vi "Filter Tester.vi"() -> ()   [LabVIEW 2016]
uses:
  Control/SSL Data Control.ctl
  Control/SSL UDP Address.ctl
  Control/File Player.ctl
  SSL/SSL Field State.ctl
  SSL Detection Frame.ctl
  SSL Detection Robot.ctl
  SSL Detection Ball.ctl
  Filters/Estimadores.ctl
  <extravilib>/ChannelInstances/Lossy Stream-t'SSL Field State.ctl'/Read With Abort.vi
  <extravilib>/ChannelInstances/Lossy Stream-a[.](u8)/Read With Abort.vi
  <extravilib>/ChannelInstances/Lossy Stream-t'SSL Field State.ctl'/Write With Abort.vi
  <extravilib>/ChannelInstances/Lossy Stream-t'SSL Field State.ctl'/Endpoint.vi
  <extravilib>/ChannelInstances/Lossy Stream-a[.](u8)/Endpoint.vi
  <extravilib>/ChannelInstances/Lossy Stream-a[.](u8)/Instantiate.vi
  <extravilib>/ChannelInstances/Lossy Stream-a[.](u8)/)Channel.vi
  <resource>/ChannelSupport/_ChannelSupport/WaitIfNeeded.vi
  <extravilib>/ChannelInstances/Lossy Stream-t'SSL Field State.ctl'/Instantiate.vi
  <extravilib>/ChannelInstances/Lossy Stream-t'SSL Field State.ctl'/)Channel.vi
  <extravilib>/ChannelInstances/Lossy Stream-t'SSL Field State.ctl'.lvlib
  <extravilib>/ChannelInstances/Lossy Stream-a[.](u8).lvlib
panel:
  out "Sinal original":sgl(graph)
  out "Ruido->Kalman":sgl(graph)
  out "Waveform Chart":sgl(graph)
  out "x^2":sgl
  out "Numeric":i32
  out "sum 3":sgl
  out "sum 2":sgl
  out "element":u8[](array[numeric])
  in  "SSL Data":T1={"Modo"=TRUE, "SSL UDP RX"={"Port:"=10020, "Server IP:"="224.5.23.2", "Local IP:"="192.168.91.173", "RX"=TRUE}, "RefBox UDP RX"={"Port:"=10021, "Server IP:"="224.5.23.2", "Local IP:"="192.168.91.173", "RX"=FALSE}, "Reprodução de Arquivo"={"file path (use dialog)"=path "E:/Media/2016-07-01_cmdragons_immortals.log", "size (in bytes)"=0, "offset (in bytes)"=0, "Slide"=0.0, "Play"=FALSE, "Time Stamp"=timestamp(0 s since 1904-01-01), "Playing"=FALSE}} {"Reprodução de Arquivo"."Time Stamp" format="%<%.3X %x>T"; "Reprodução de Arquivo"."Slide" min=0 max=1 scale=0.0..1.0; "Reprodução de Arquivo"."offset (in bytes)" format="%.3p"; "Reprodução de Arquivo"."size (in bytes)" format="%.3p"}
  # "UDP"
  # "LOG"
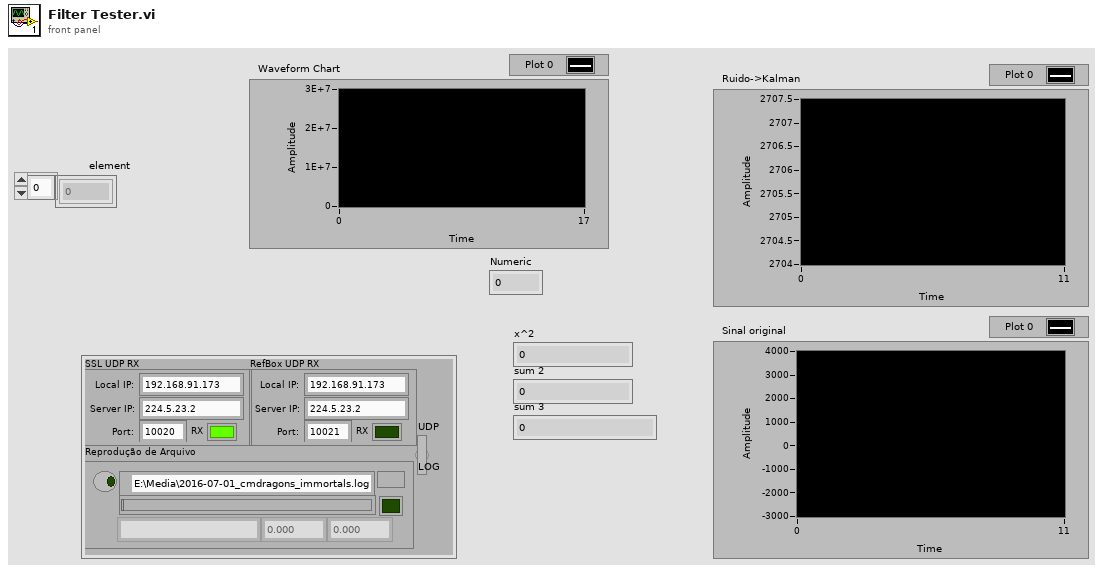
[diagram p1: front panel]
types:
  T1 = typedef "SSL Data Control.ctl" = cluster{"Modo":bool, "SSL UDP RX":T2, "RefBox UDP RX":T2, "Reprodução de Arquivo":T3}
  T2 = typedef "SSL UDP Address.ctl" = cluster{"Port:":u16, "Server IP:":string, "Local IP:":string, "RX":bool}
  T3 = typedef "File Player.ctl" = cluster{"file path (use dialog)":path, "size (in bytes)":i64, "offset (in bytes)":i64, "Slide":sgl, "Play":bool, "Time Stamp":timestamp, "Playing":bool}
  T4 = typedef "Lossy Stream-a[.](u8).lvlib/)Channel.ctl" = refnum<queue>
  T5 = typedef "Estimadores.ctl" = enum16{"Nenhum", "Simples", "Simples Timestamp", "Simples Mult Cam", "Kalman", "Kalman Mult Cam"}
  T6 = typedef "SSL Field State.ctl" = cluster{"Detection Frame Out":T7, "Field Size Out":cluster{"line_width":u32, "field_length":u32, "field_width":u32, "boundary_width":u32, "referee_width":u32, "goal_width":u32, "goal_depth":u32, "goal_wall_width":u32, "center_circle_radius":u32, "defense_radius":u32, "defense_stretch":u32, "free_kick_from_defense_dist":u32, "penalty_spot_from_field_line_dist":u32, "penalty_line_from_spot_dist":u32}, "Received Time Stamp":timestamp}
  T7 = typedef "SSL Detection Frame.ctl" = cluster{"frame_number":u32, "t_capture":dbl, "t_sent":dbl, "camera_id":u32, "robots_yellow":T8[], "robots_blue":T8[], "balls":T9[], "Valid":bool, "Time Stamp":timestamp}
  T8 = typedef "SSL Detection Robot.ctl" = cluster{"x":sgl, "robot_id":u32, "confidence":sgl, "y":sgl, "orientation":sgl, "pixel_x":sgl, "pixel_y":sgl, "height":sgl, "Valid":bool, "Time Stamp":timestamp}
  T9 = typedef "SSL Detection Ball.ctl" = cluster{"x":sgl, "area":u32, "confidence":sgl, "y":sgl, "z":sgl, "pixel_x":sgl, "pixel_y":sgl, "Valid":bool, "Time Stamp":timestamp}
  T10 = cluster{"line_width":u32, "field_length":u32, "field_width":u32, "boundary_width":u32, "referee_width":u32, "goal_width":u32, "goal_depth":u32, "goal_wall_width":u32, "center_circle_radius":u32, "defense_radius":u32, "defense_stretch":u32, "free_kick_from_defense_dist":u32, "penalty_spot_from_field_line_dist":u32, "penalty_line_from_spot_dist":u32}
  T11 = typedef "Lossy Stream-t'SSL Field State.ctl'.lvlib/)Channel.ctl" = refnum<queue>
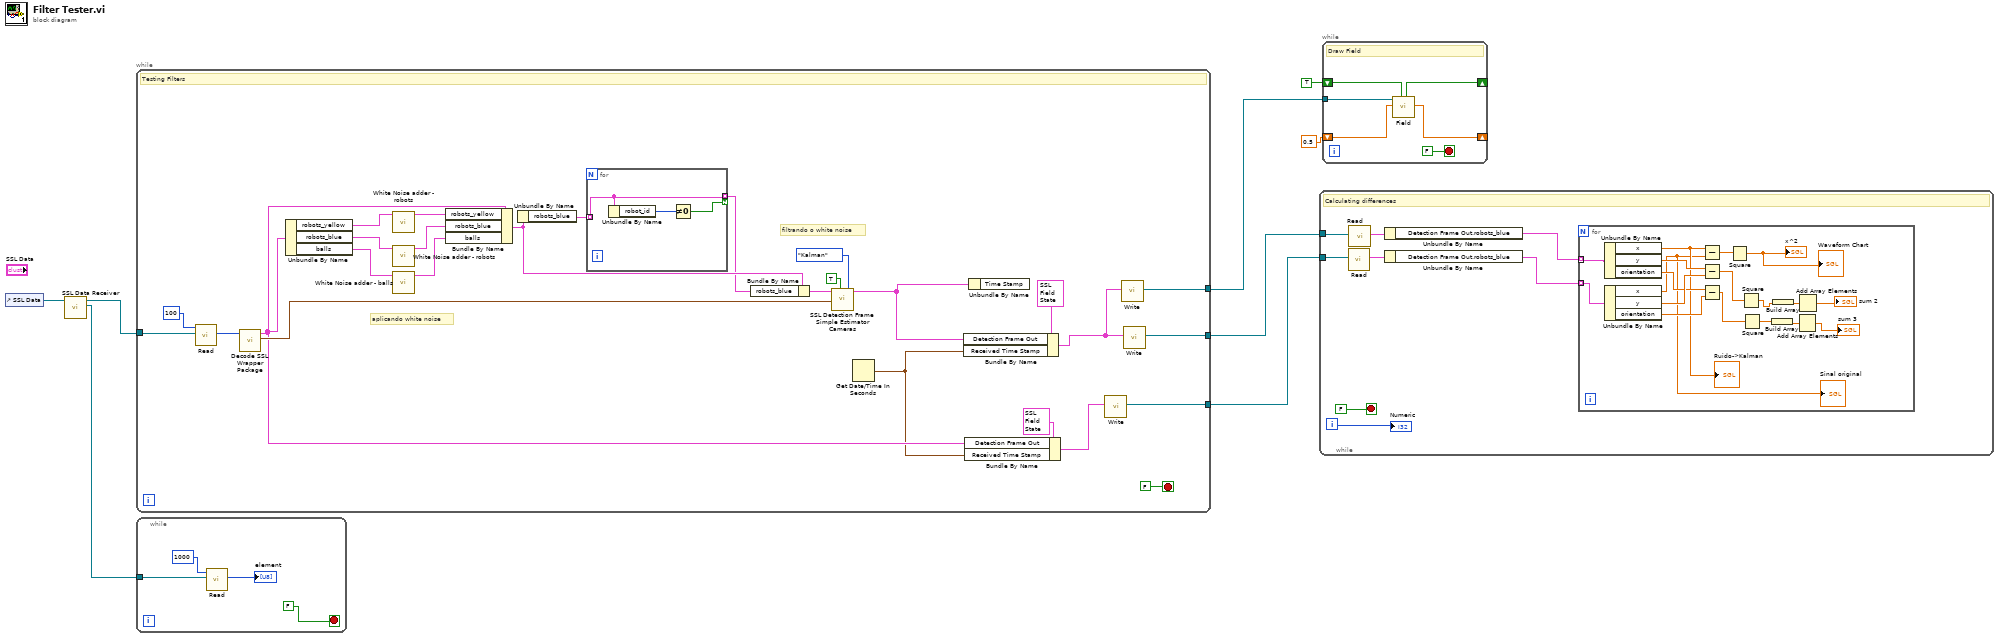
[diagram p0: block diagram]
diagram:
  n1 = control-ref of="SSL Data"() -> (w8:refnum<vi>)
  n2 = call "SSL Data Receiver.vi"("SSL Data 2"=w8) -> ("SSL RefBox"=w1:T4, "SSL Vision"=w4:T4)  [unwired: 9 in]
  n3 = while {
    tunnel: [w31] -> w5
    tunnel: w4 -> [w28]
    tunnel: [w15] -> w3
    tunnel: [w14] -> w2
    stop <- FALSE stop-if-true
    # "filtrando o white noise"
    # "aplicando white noise"
    # "Testing Filters"
    n4 = call <extravilib>:"Read.vi"("channel"=w28, "timeout in ms (-1)"=100) -> ("element"=w27:u8[])  [unwired: 4 in, 5 out]
    n5 = call "Decode SSL Wrapper Package.vi"("unsigned byte array"=w27) -> ("Field Size"=w34:T10, "Detection Frame"=w21:T7)  [unwired: 7 in, 2 out]
    n6 = Unbundle By Name(w21) -> ("robots_yellow"=w24:T8[], "robots_blue"=w23:T8[], "balls"=w22:T9[])
    n7 = call "White Noise adder - robots.vi"("robots"=w24) -> ("Robots w noise"=w20:T8[])  [unwired: 8 in]
    n8 = call "White Noise adder - robots.vi"("robots"=w23) -> ("Robots w noise"=w19:T8[])  [unwired: 8 in]
    n9 = call "White Noise adder - balls.vi"("balls"=w22) -> ("balls w/ noise"=w18:T9[])  [unwired: 8 in]
    n10 = Bundle By Name(cluster=w21, "robots_yellow"=w20, "robots_blue"=w19, "balls"=w18) -> (w12:T7)
    n11 = Unbundle By Name(w12) -> ("robots_blue"=w13:T8[])
    n12 = for {
      tunnel: w13 -> [w38] mode=indexing
      tunnel: [w38] -> w10 mode=indexing if=w36
      n13 = Unbundle By Name(w38) -> ("robot_id"=w37:u32)
      n14 = Not Equal To 0?(x=w37) -> (x != 0?=w36:bool)
    }
    n15 = Bundle By Name(cluster=w12, "robots_blue"=w10) -> (w11:T7)
    n16 = call "SSL Detection Frame Simple Estimator Cameras.vi"("Estimador"=Estimadores."Kalman", "Enable"=TRUE, "Field Size"=w34, "Detection Frame In"=w11) -> ("Detection Frame Out"=w9:T7)  [unwired: 6 in, 1 out]
    n17 = Get Date/Time In Seconds() -> (seconds since 1Jan1904=w17:timestamp)
    n18 = Bundle By Name(cluster=T6 {"Detection Frame Out"={"frame_number"=0, "t_capture"=0.0, "t_sent"=0.0, "camera_id"=0, "robots_yellow"=[], "robots_blue"=[], "balls"=[], "Valid"=FALSE, "Time Stamp"=timestamp(0 s since 1904-01-01)}, "Field Size Out"={"line_width"=0, "field_length"=0, "field_width"=0, "boundary_width"=0, "referee_width"=0, "goal_width"=0, "goal_depth"=0, "goal_wall_width"=0, "center_circle_radius"=0, "defense_radius"=0, "defense_stretch"=0, "free_kick_from_defense_dist"=0, "penalty_spot_from_field_line_dist"=0, "penalty_line_from_spot_dist"=0}, "Received Time Stamp"=timestamp(0 s since 1904-01-01)}, "Detection Frame Out"=w9, "Received Time Stamp"=w17) -> (w30:T6)
    n19 = Bundle By Name(cluster=T6 {"Detection Frame Out"={"frame_number"=0, "t_capture"=0.0, "t_sent"=0.0, "camera_id"=0, "robots_yellow"=[], "robots_blue"=[], "balls"=[], "Valid"=FALSE, "Time Stamp"=timestamp(0 s since 1904-01-01)}, "Field Size Out"={"line_width"=0, "field_length"=0, "field_width"=0, "boundary_width"=0, "referee_width"=0, "goal_width"=0, "goal_depth"=0, "goal_wall_width"=0, "center_circle_radius"=0, "defense_radius"=0, "defense_stretch"=0, "free_kick_from_defense_dist"=0, "penalty_spot_from_field_line_dist"=0, "penalty_line_from_spot_dist"=0}, "Received Time Stamp"=timestamp(0 s since 1904-01-01)}, "Detection Frame Out"=w21, "Received Time Stamp"=w17) -> (w16:T6)
    n20 = Unbundle By Name(w9) -> ()  [unwired: 1 out]
    n21 = call <extravilib>:"Write.vi"("element"=w16) -> ("channel"=w15:T11)  [unwired: 8 in, 2 out]
    n22 = call <extravilib>:"Write.vi"("element"=w30) -> ("channel"=w31:T11)  [unwired: 8 in, 2 out]
    n23 = call <extravilib>:"Write.vi"("element"=w30) -> ("channel"=w14:T11)  [unwired: 8 in, 2 out]
  }
  n24 = while {
    tunnel: w1 -> [w40]
    stop <- FALSE stop-if-true
    n25 = call <extravilib>:"Read.vi"("channel"=w40, "timeout in ms (-1)"=1000) -> ("element"=→"element":u8[])  [unwired: 4 in, 5 out]
  }
  n26 = while {
    tunnel: w3 -> [w49]
    tunnel: w2 -> [w50]
    i -> [w43]
    stop <- FALSE stop-if-true
    # "Calculating differences"
    n27 = call <extravilib>:"Read.vi"("channel"=w49) -> ("element"=w47:T6)  [unwired: 5 in, 5 out]
    n28 = call <extravilib>:"Read.vi"("channel"=w50) -> ("element"=w48:T6)  [unwired: 5 in, 5 out]
    n29 = Unbundle By Name(w48) -> ("Detection Frame Out.robots_blue"=w46:T8[])
    n30 = Unbundle By Name(w47) -> ("Detection Frame Out.robots_blue"=w45:T8[])
    n31 = for {
      tunnel: w46 -> [w68] mode=indexing
      tunnel: w45 -> [w67] mode=indexing
      n32 = Unbundle By Name(w68) -> ("x"=w52:sgl, "y"=w66:sgl, "orientation"=w64:sgl)
      "Ruido->Kalman" <- w52
      n33 = Unbundle By Name(w67) -> ("x"=w51:sgl, "y"=w65:sgl, "orientation"=w63:sgl)
      "Sinal original" <- w51
      n34 = Subtract(x=w52, y=w51) -> (x-y=w62:sgl)
      n35 = Subtract(x=w66, y=w65) -> (x-y=w61:sgl)
      n36 = Subtract(x=w64, y=w63) -> (x-y=w60:sgl)
      n37 = Square(x=w62) -> (x^2=→"x^2" →"Waveform Chart":sgl)
      n38 = Square(x=w61) -> (x^2=w57:sgl)
      n39 = Square(x=w60) -> (x^2=w56:sgl)
      n40 = Build Array(w56) -> (w58:sgl[])
      n41 = Build Array(w57) -> (w59:sgl[])
      n42 = Add Array Elements(numeric array=w58) -> (sum=→"sum 3":sgl)
      n43 = Add Array Elements(numeric array=w59) -> (sum=→"sum 2":sgl)
    }
    "Numeric" <- w43
  }
  n44 = while {
    shift-right: [w72] -> _
    shift-left: 0.5 ("New Scale") -> [w74]
    shift-right: [w71] -> _
    shift-left: TRUE ("AutoScale Out") -> [w70]
    tunnel: w5 -> [w69]
    stop <- FALSE stop-if-true
    # "Draw Field"
    n45 = call "Field.vi"("AutoScale"=w70, "Scale mm/pixel"=w74, "channel"=w69) -> ("Scale Out"=w72:dbl, "AutoScale Out"=w71:bool)  [unwired: 6 in, 1 out]
  }
